vi "Count60_2Ch.vi"(6 "Last samples in":T1, 8 "Count type":bool=TRUE, 9 "Area interloop cluster":T2, 10 "Photon counters area 2 in":cluster{u16, u16}, 11 "Photon counters area 1 in":cluster{u16, u16}) -> (2 "Photon counters area 2 out":cluster{u16, u16}, 3 "Photon counters area 1 out":cluster{u16, u16}, 4 "New last samples out":T1)   [LabVIEW 2012]
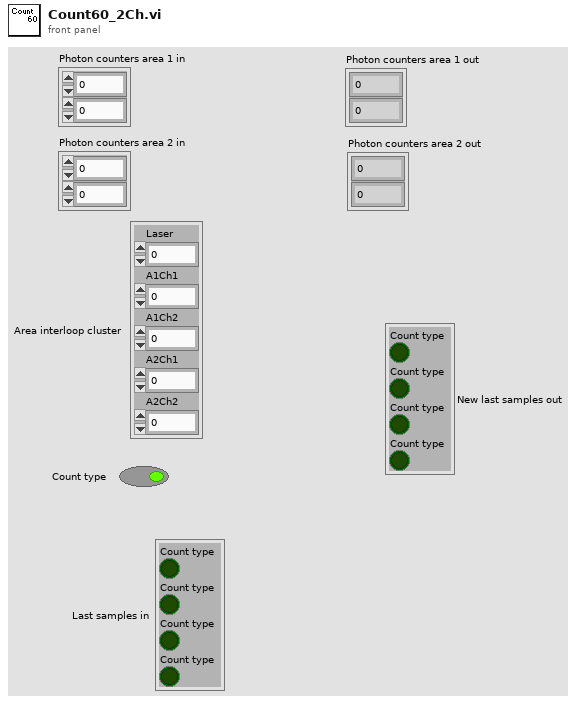
[diagram p1: front panel]
types:
  T1 = cluster{"Count type":bool, "Count type":bool, "Count type":bool, "Count type":bool}
  T2 = cluster{"Laser":u64, "A1Ch1":u64, "A1Ch2":u64, "A2Ch1":u64, "A2Ch2":u64}
  T3 = cluster{"New high count":u16, "New high count":u16}
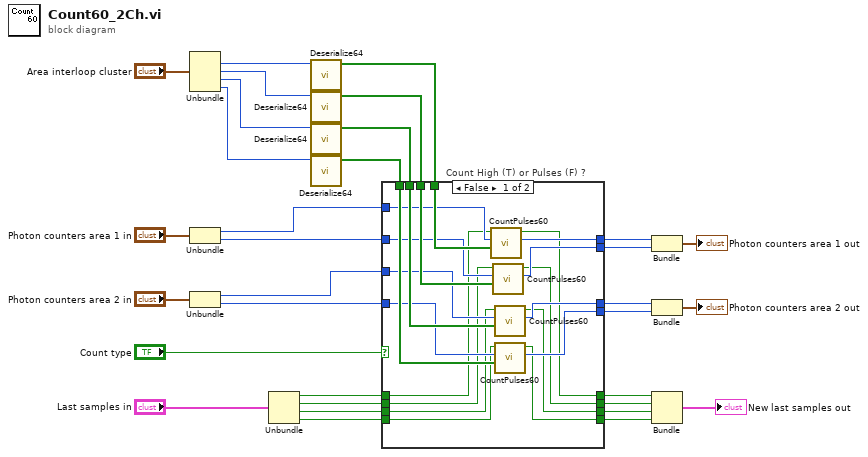
[diagram p0: block diagram]
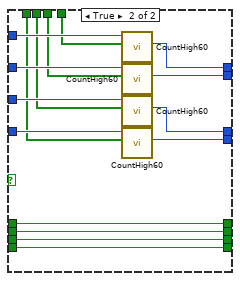
[diagram p2: hidden frame]
diagram:
  n1 = Unbundle("Area interloop cluster") -> ("A1Ch1"=w12:u64, "A1Ch2"=w13:u64, "A2Ch1"=w14:u64, "A2Ch2"=w15:u64)  [unwired: 1 out]
  n2 = Unbundle("Photon counters area 1 in") -> (w30:u16, w28:u16)
  n3 = Unbundle("Photon counters area 2 in") -> (w29:u16, w27:u16)
  n4 = Unbundle("Last samples in") -> ("Count type"=w9:bool, "Count type"=w8:bool, "Count type"=w7:bool, "Count type"=w6:bool)
  n5 = call "Deserialize64.vi"("U64 input"=w12) -> ("60bit output"=w20:bool[])  [unwired: 10 in]
  n6 = call "Deserialize64.vi"("U64 input"=w13) -> ("60bit output"=w19:bool[])  [unwired: 10 in]
  n7 = call "Deserialize64.vi"("U64 input"=w14) -> ("60bit output"=w18:bool[])  [unwired: 10 in]
  n8 = call "Deserialize64.vi"("U64 input"=w15) -> ("60bit output"=w17:bool[])  [unwired: 10 in]
  n9 = case "Count High (T) or Pulses (F) ?" shown="False" "Count type" {
    tunnel: w30 -> [w46 w68]
    tunnel: w29 -> [w44 w67]
    tunnel: w28 -> [w45 w66]
    tunnel: w27 -> [w43 w65]
    tunnel: [w51 w64] -> w26
    tunnel: [w49 w63] -> w25
    tunnel: [w42 w62] -> w24
    tunnel: [w41 w61] -> w23
    tunnel: w20 -> [w52 w60]
    tunnel: w19 -> [w50 w59]
    tunnel: w18 -> [w48 w58]
    tunnel: w17 -> [w47 w57]
    tunnel: w9 -> [w40 w56]
    tunnel: w8 -> [w39 w55]
    tunnel: w7 -> [w38 w54]
    tunnel: w6 -> [w37 w53]
    tunnel: [w36 w56] -> w5
    tunnel: [w35 w55] -> w4
    tunnel: [w34 w54] -> w3
    tunnel: [w33 w53] -> w2
    frame False {
      n10 = call "CountPulses60.vi"("60bit input"=w52, "Previous pulse count"=w46, "Last sample"=w40) -> ("New pulse count"=w51:u16, "New last sample"=w36:bool)  [unwired: 7 in]
      n11 = call "CountPulses60.vi"("60bit input"=w50, "Previous pulse count"=w45, "Last sample"=w39) -> ("New pulse count"=w49:u16, "New last sample"=w35:bool)  [unwired: 7 in]
      n12 = call "CountPulses60.vi"("60bit input"=w48, "Previous pulse count"=w44, "Last sample"=w38) -> ("New pulse count"=w42:u16, "New last sample"=w34:bool)  [unwired: 7 in]
      n13 = call "CountPulses60.vi"("60bit input"=w47, "Previous pulse count"=w43, "Last sample"=w37) -> ("New pulse count"=w41:u16, "New last sample"=w33:bool)  [unwired: 7 in]
    }
    frame True {
      n14 = call "CountHigh60.vi"("60bit input"=w60, "Previous high count"=w68) -> ("New high count"=w64:u16)  [unwired: 9 in]
      n15 = call "CountHigh60.vi"("60bit input"=w59, "Previous high count"=w66) -> ("New high count"=w63:u16)  [unwired: 9 in]
      n16 = call "CountHigh60.vi"("60bit input"=w58, "Previous high count"=w67) -> ("New high count"=w62:u16)  [unwired: 9 in]
      n17 = call "CountHigh60.vi"("60bit input"=w57, "Previous high count"=w65) -> ("New high count"=w61:u16)  [unwired: 9 in]
    }
  }
  n18 = Bundle("New high count"=w26, "New high count"=w25) -> (→"Photon counters area 1 out":T3)  [unwired: 1 in]
  n19 = Bundle("New high count"=w24, "New high count"=w23) -> (→"Photon counters area 2 out":T3)  [unwired: 1 in]
  n20 = Bundle("Count type"=w5, "Count type"=w4, "Count type"=w3, "Count type"=w2) -> (→"New last samples out":T1)  [unwired: 1 in]
